vi "TimeQueue.vi"() -> (0 "error out":errorcluster, 3 "Queue out":refnum<queue>)   [LabVIEW 2018]
doc: "Crea la coda di messaggi per la comunicazione con il timer."
uses:
  TimeCluster.ctl
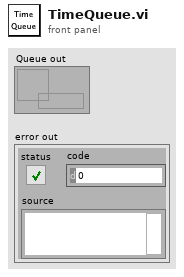
[diagram p1: front panel]
types:
  T1 = typedef "TimeCluster.ctl" = cluster{"run":bool, "destroy":bool, "Elapsed time":i32, "WaitTime":i32, "Ticktime":i32}
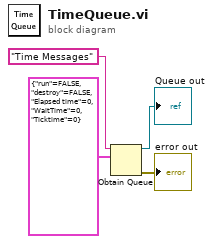
[diagram p0: block diagram]
diagram:
  n1 = Obtain Queue(name (unnamed)="Time Messages", element data type=T1 {"run"=FALSE, "destroy"=FALSE, "Elapsed time"=0, "WaitTime"=0, "Ticktime"=0}) -> (queue out=→"Queue out":refnum<queue>, error out=→"error out":errorcluster)  [unwired: 3 in, 1 out]
